vi "Check DAQ Sensors.vi"(8 "error in (no error)":errorcluster, 11 "Test Type":string) -> (0 "error out":errorcluster, 1 "Errors":errorcluster[](array[cluster]), 2 "Oil Present?":bool, 3 "H2 Not Ready?":bool, 5 "Error?":bool)   [LabVIEW 2014]
uses:
  CAN Communication/PAS/PAS.lvclass
  CAN Communication/PAS/Typedefs/Pressure Sensor.ctl
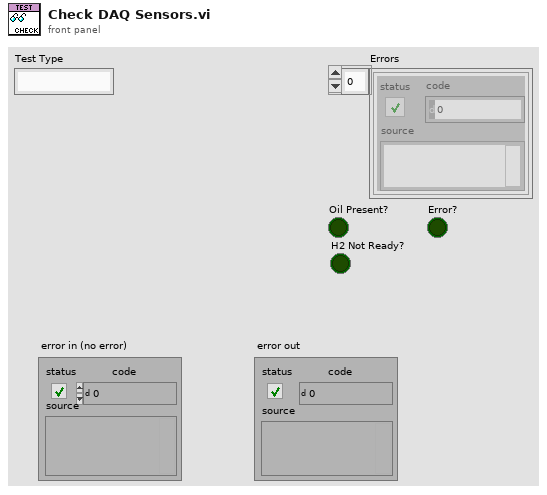
[diagram p1: front panel]
types:
  T1 = typedef "PAS.lvclass/Pressure Sensor.ctl" = u16
  T2 = typedef "PAS.lvclass/Session Handle.ctl" = refnum<data-value>
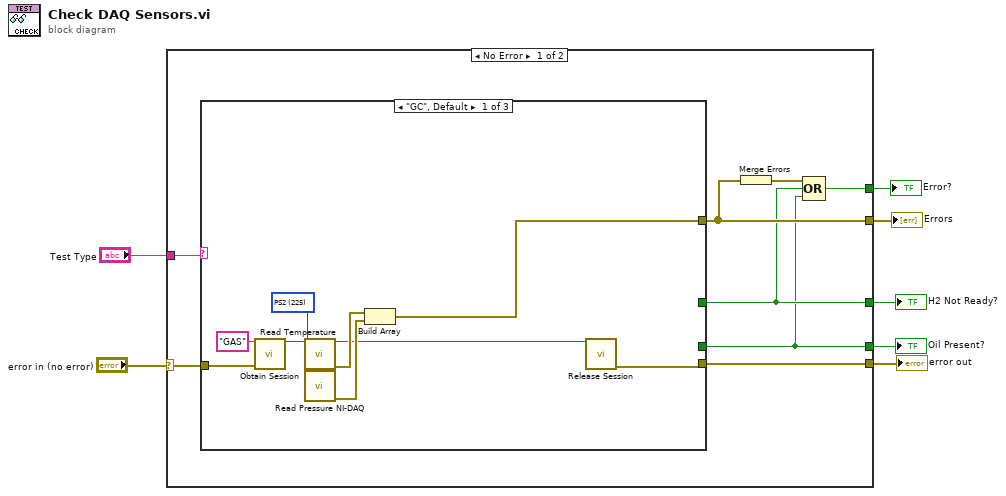
[diagram p0: block diagram]
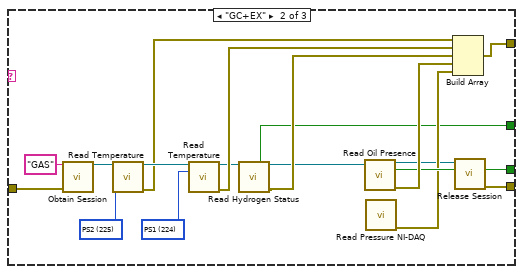
[diagram p2: hidden frame]
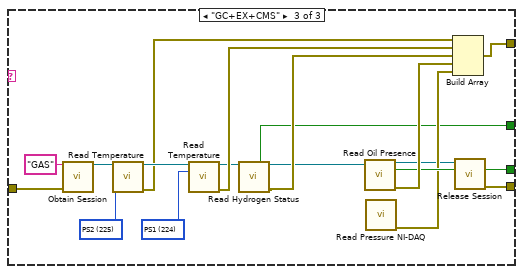
[diagram p3: hidden frame]
diagram:
  n1 = case shown="No Error" "error in (no error)" {
    selector: "error in (no error)" -> [w14 w61]
    tunnel: "Test Type" -> [w15 _]
    tunnel: [w12 _] -> w5
    tunnel: [w9 _] -> w4
    tunnel: [w13 w61] -> w3
    tunnel: [w10 _] -> w2
    tunnel: [w8 _] -> w1
    frame No Error {
      n2 = case shown="\"GC\", Default" w15 {
        tunnel: w14 -> [w23 w41 w59]
        tunnel: [w18 w38 w56] -> w12
        tunnel: [_ w32 w50] -> w9
        tunnel: [w16 w29 w47] -> w13
        tunnel: [_ w25 w43] -> w10
        frame "GC", Default {
          w22 = T1 225 items=["PS1"=224, "PS2"=225] ("Pressure Sensor")
          n3 = call "Obtain Session.vi"("Session  Name ()"="GAS", "error in (no error)"=w23) -> ("Session Handle"=w21:T2)  [unwired: 12 in, 1 out]
          n4 = call "Read Temperature.vi"("Session Handle in"=w21, 5:w22) -> ("Session Handle out"=w17:T2, "error out"=w20:errorcluster)  [unwired: 9 in, 3 out]
          n5 = call "Read Pressure NI-DAQ.vi"() -> ("error out"=w19:errorcluster)  [unwired: 10 in, 1 out]
          n6 = Build Array(w20, w19) -> (w18:errorcluster[])
          n7 = call "Release Session.vi"("Session Handle"=w17) -> ("error out"=w16:errorcluster)  [unwired: 14 in]
        }
        frame "GC+EX" {
          w36 = T1 224 items=["PS1"=224, "PS2"=225] ("Pressure Sensor")
          w40 = T1 225 items=["PS1"=224, "PS2"=225] ("Pressure Sensor")
          n8 = call "Obtain Session.vi"("Session  Name ()"="GAS", "error in (no error)"=w41) -> ("Session Handle"=w39:T2)  [unwired: 12 in, 1 out]
          n9 = call "Read Temperature.vi"("Session Handle in"=w39, 5:w40) -> ("Session Handle out"=w37:T2, "error out"=w35:errorcluster)  [unwired: 9 in, 3 out]
          n10 = call "Read Temperature.vi"("Session Handle in"=w37, 5:w36) -> ("Session Handle out"=w28:T2, "error out"=w34:errorcluster)  [unwired: 9 in, 3 out]
          n11 = call "Read Hydrogen Status.vi"("Session Handle in"=w28) -> ("Ready?"=w25:bool, "Session Handle out"=w26:T2, "error out"=w27:errorcluster)  [unwired: 9 in, 3 out]
          n12 = call "Read Oil Presence.vi"("Session Handle in"=w26) -> ("Session Handle out"=w30:T2, "Present?"=w32:bool, "error out"=w33:errorcluster)  [unwired: 12 in]
          n13 = call "Read Pressure NI-DAQ.vi"() -> ("error out"=w31:errorcluster)  [unwired: 10 in, 1 out]
          n14 = Build Array(w35, w34, w27, w33, w31) -> (w38:errorcluster[])
          n15 = call "Release Session.vi"("Session Handle"=w30) -> ("error out"=w29:errorcluster)  [unwired: 14 in]
        }
        frame "GC+EX+CMS" {
          w54 = T1 224 items=["PS1"=224, "PS2"=225] ("Pressure Sensor")
          w58 = T1 225 items=["PS1"=224, "PS2"=225] ("Pressure Sensor")
          n16 = call "Obtain Session.vi"("Session  Name ()"="GAS", "error in (no error)"=w59) -> ("Session Handle"=w57:T2)  [unwired: 12 in, 1 out]
          n17 = call "Read Temperature.vi"("Session Handle in"=w57, 5:w58) -> ("Session Handle out"=w55:T2, "error out"=w53:errorcluster)  [unwired: 9 in, 3 out]
          n18 = call "Read Temperature.vi"("Session Handle in"=w55, 5:w54) -> ("Session Handle out"=w46:T2, "error out"=w52:errorcluster)  [unwired: 9 in, 3 out]
          n19 = call "Read Hydrogen Status.vi"("Session Handle in"=w46) -> ("Ready?"=w43:bool, "Session Handle out"=w44:T2, "error out"=w45:errorcluster)  [unwired: 9 in, 3 out]
          n20 = call "Read Oil Presence.vi"("Session Handle in"=w44) -> ("Session Handle out"=w48:T2, "Present?"=w50:bool, "error out"=w51:errorcluster)  [unwired: 12 in]
          n21 = call "Read Pressure NI-DAQ.vi"() -> ("error out"=w49:errorcluster)  [unwired: 10 in, 1 out]
          n22 = Build Array(w53, w52, w45, w51, w49) -> (w56:errorcluster[])
          n23 = call "Release Session.vi"("Session Handle"=w48) -> ("error out"=w47:errorcluster)  [unwired: 14 in]
        }
      }
      n24 = Merge Errors(w12) -> (w11:errorcluster)
      n25 = Compound Arithmetic op=OR(w11, w10, w9) -> (w8:bool)
    }
    frame Error {
    }
  }
  "error out" <- w3
  "Errors" <- w5
  "Oil Present?" <- w4
  "H2 Not Ready?" <- w2
  "Error?" <- w1
